vi "CRYReport Part ObjectZoomed Event Callback.vi"(4 "TXTextControl":refnum<k7>, 6 "Control Ref":refnum<k7>, 7 "Event Common Data":T1) -> ()   [LabVIEW 2013]
uses:
  CRYReport Global.vi
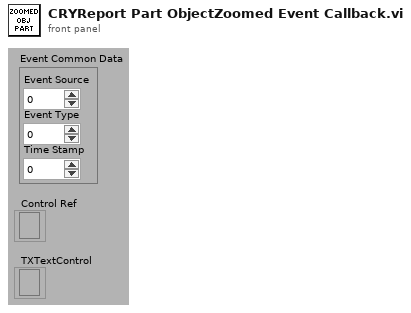
[diagram p1: front panel]
types:
  T1 = cluster{"Event Source":i32, "Event Type":u32, "Time Stamp":u32}
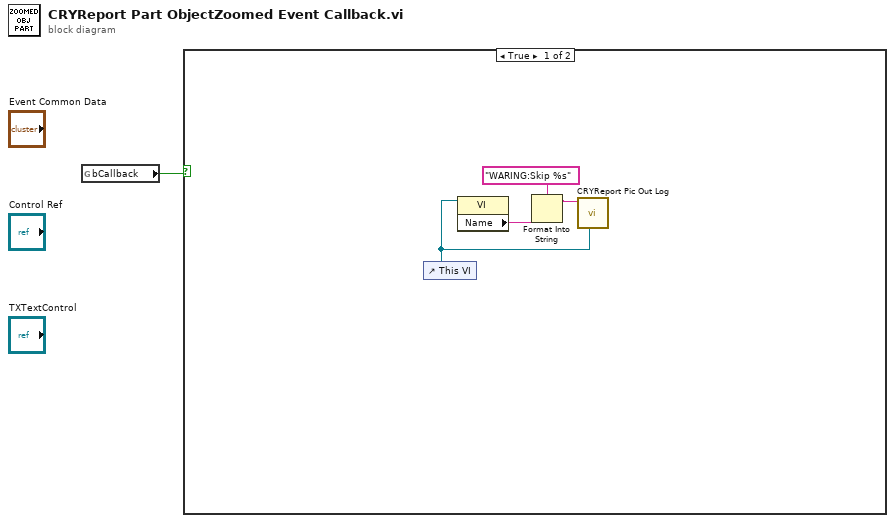
[diagram p0: block diagram]
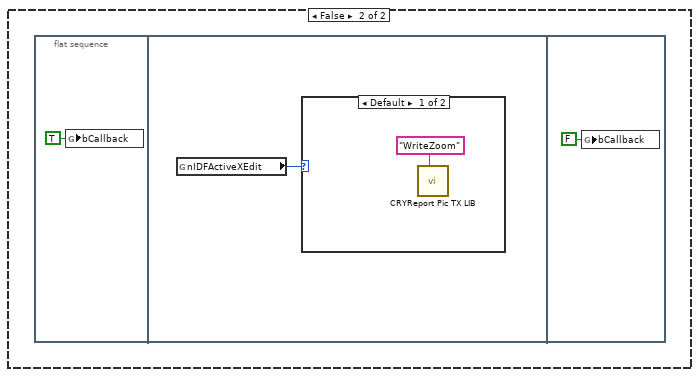
[diagram p2: hidden frame]
diagram:
  n1 = global read "CRYReport Global.vi" "bCallback"() -> (w1:bool)
  n2 = case shown="True" w1 {
    frame True {
      n3 = control-ref of="This VI"() -> (w2:refnum<vi>)
      n4 = property class="VI"(reference=w2) -> ("Name"=w3:string)  [unwired: 1 in, 2 out]
      n5 = Format Into String(format string="WARING:Skip %s" ("string"), w3) -> (resulting string=w5:string)  [unwired: 2 in, 1 out]
      n6 = call "CRYReport Pic Out Log.vi"("vi reference"=w2, "sData"=w5) -> ()  [unwired: 10 in]
    }
    frame False {
      n7 = flat-sequence {
        frame #0 {
          n8 = global write "CRYReport Global.vi" "bCallback"(TRUE ("bCallback")) -> ()
        }
        frame #1 {
          n9 = global read "CRYReport Global.vi" "nIDFActiveXEdit"() -> (w7:i16)
          n10 = case shown="Default" w7 {
            frame Default {
              n11 = call "CRYReport Pic TX LIB.vi"("sAction"="WriteZoom") -> ()  [unwired: 8 in, 3 out]
            }
            frame -1 {
            }
          }
        }
        frame #2 {
          n12 = global write "CRYReport Global.vi" "bCallback"(FALSE ("bCallback")) -> ()
        }
      }
    }
  }
